vi "Formic Queen.vi"(8 "error in (no error)":errorcluster, 9 "SelfID":i32, 10 "Map":i32[](array[numeric]), 11 "Mother in":refnum<class "Formics.lvclass">) -> (0 "error out":errorcluster, 1 "Direction":T1, 2 "Action":T2, 3 "Mother out":refnum<class "Formics.lvclass">, 4 "Replicated Class":refnum<class "Formics.lvclass">)   [LabVIEW 2015, in "Formics.lvclass"]
uses:
  Formics.lvclass
  Type Defs/Action Enum.ctl
  Type Defs/Direction Enum.ctl
  Formics.lvclass/Formics.ctl
  SquareStatus.ctl
  Formic Types.ctl
  Kamikaze DVR Cluster.ctl
  Type Defs/SB Type Defs.lvlib
  Common/Common.lvlib
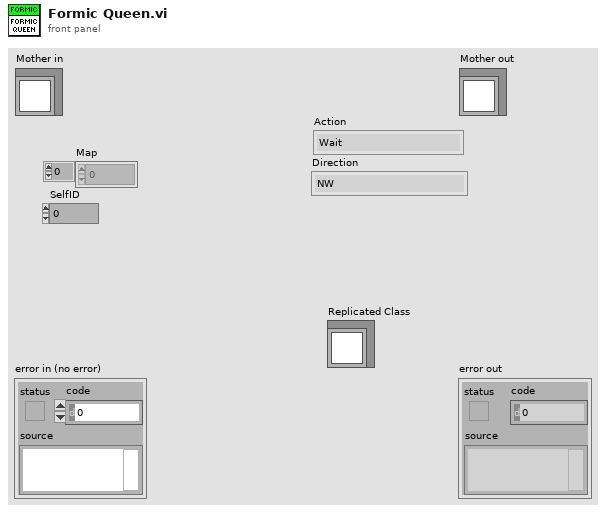
[diagram p1: front panel]
types:
  T1 = typedef "SB Type Defs.lvlib/Direction Enum.ctl" = enum16{"NW", "N", "NE", "E", "SE", "S", "SW", "W"}
  T2 = typedef "SB Type Defs.lvlib/Action Enum.ctl" = enum16{"Wait", "Move", "Attack", "Replicate"}
  T3 = typedef "Kamikaze DVR Cluster.ctl" = cluster{"Kamikaze?":bool, "Direction":u8}
  T4 = typedef "Formics.lvclass/Formic Types.ctl" = enum16{"Queen Bee", "Protector Bee", "Daughter Bee", "Worker Bee", "Coward"}
  T5 = typedef "Formics.lvclass/SquareStatus.ctl" = cluster{"ID":i32, "Heartbeat":bool, "MyPosition":cluster{"X":i32, "Y":i32}}
  T6 = typedef "Formics.lvclass/Kamikaze DVR.ctl" = refnum<data-value>
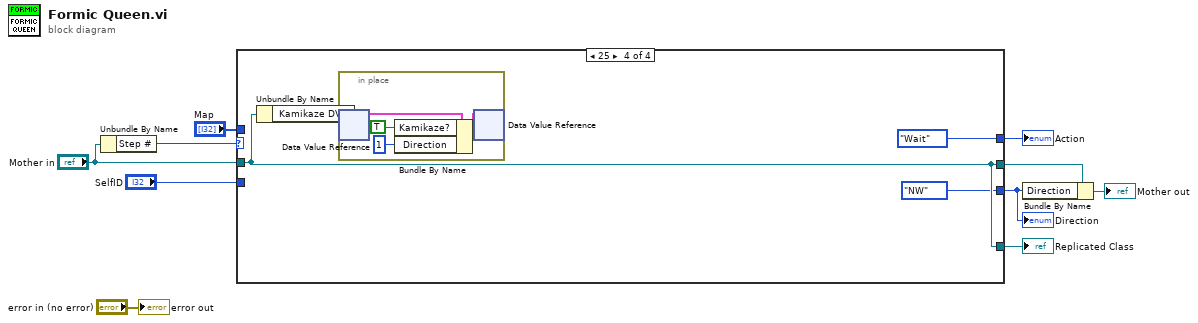
[diagram p0: block diagram]
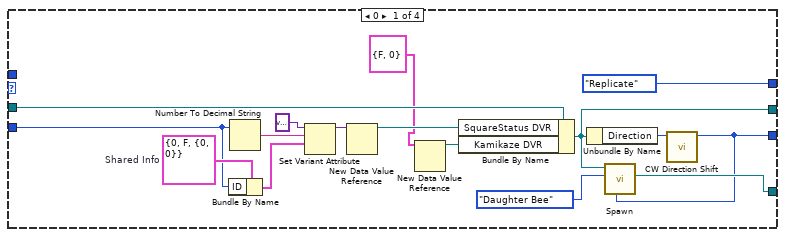
[diagram p2: hidden frame]
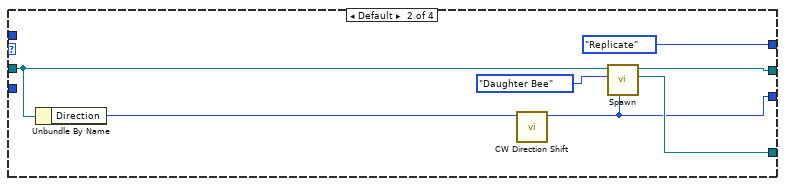
[diagram p3: hidden frame]
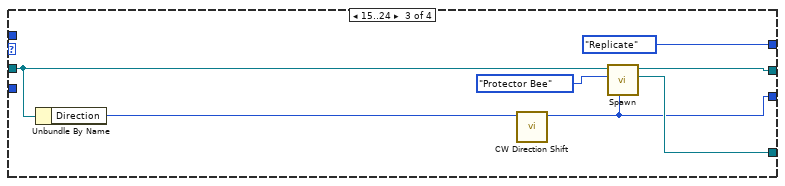
[diagram p4: hidden frame]
diagram:
  n1 = Unbundle By Name("Mother in") -> ("Step #"=w7:i32)
  n2 = case shown="25" w7 {
    tunnel: [w15 w29 w36 w42] -> w9
    tunnel: "Mother in" -> [w20 w30 w37 w42]
    tunnel: "SelfID" -> [w19 _ _ _]
    tunnel: "Map" -> [_ _ _ _]
    tunnel: [Action_Enum."Replicate" ("Action") Action_Enum."Replicate" ("Action") Action_Enum."Replicate" ("Action") Action_Enum."Wait" ("Action")] -> w4
    tunnel: [w14 w28 w35 Direction_Enum."NW" ("Direction")] -> w1
    tunnel: [w17 w31 w38 w42] -> w3
    frame 0 {
      w24 = T5 {"ID"=0, "Heartbeat"=FALSE, "MyPosition"={"X"=0, "Y"=0}}  # Shared Info
      n3 = Bundle By Name(cluster=w24, "ID"=w19) -> (w25:T5)
      n4 = Number To Decimal String(number=w19) -> (decimal integer string=w26:string)  [unwired: 1 in]
      n5 = Set Variant Attribute(Variant=variant ("variant"), name=w26, value=w25) -> (Variant out=w23:variant)  [unwired: 1 in, 2 out]
      n6 = New Data Value Reference(data value=w23) -> (data value reference=w22:refnum<data-value>)  [unwired: 1 in, 1 out]
      n7 = New Data Value Reference(data value=T3 {"Kamikaze?"=FALSE, "Direction"=0}) -> (data value reference=w11:refnum<data-value>)  [unwired: 1 in, 1 out]
      n8 = Bundle By Name(cluster=w20, "SquareStatus DVR"=w22, "Kamikaze DVR"=w11) -> (w15:refnum<class "Formics.lvclass">)
      n9 = Unbundle By Name(w15) -> ("Direction"=w13:i32)
      n10 = call "CW Direction Shift.vi"("Direction"=w13) -> ("Numeric"=w14:i32)  [unwired: 10 in]
      n11 = call "Spawn.vi"("Start Direction"=w14, "Directive"=Formic_Types."Daughter Bee", "Mother in"=w15) -> ("Replicated Class"=w17:refnum<class "Formics.lvclass">)  [unwired: 6 in, 2 out]
    }
    frame Default {
      n12 = Unbundle By Name(w30) -> ("Direction"=w27:i32)
      n13 = call "CW Direction Shift.vi"("Direction"=w27) -> ("Numeric"=w28:i32)  [unwired: 10 in]
      n14 = call "Spawn.vi"("Start Direction"=w28, "Directive"=Formic_Types."Daughter Bee", "Mother in"=w30) -> ("Replicated Class"=w31:refnum<class "Formics.lvclass">, "Mother out"=w29:refnum<class "Formics.lvclass">)  [unwired: 6 in, 1 out]
    }
    frame 15..24 {
      n15 = Unbundle By Name(w37) -> ("Direction"=w34:i32)
      n16 = call "CW Direction Shift.vi"("Direction"=w34) -> ("Numeric"=w35:i32)  [unwired: 10 in]
      n17 = call "Spawn.vi"("Start Direction"=w35, "Directive"=Formic_Types."Protector Bee", "Mother in"=w37) -> ("Replicated Class"=w38:refnum<class "Formics.lvclass">, "Mother out"=w36:refnum<class "Formics.lvclass">)  [unwired: 6 in, 1 out]
    }
    frame 25 {
      n18 = Unbundle By Name(w42) -> ("Kamikaze DVR"=w44:T6)
      n19 = in-place {
        n20 = in-place-dvr #1(w44) -> (w48:T3)  [unwired: 1 out]
        n21 = Bundle By Name(cluster=w48, "Kamikaze?"=TRUE, "Direction"=u8 1) -> (w47:T3)
        n22 = in-place-dvr #1(w47) -> ()  [unwired: 2 out]
      }
    }
  }
  "Action" <- w4
  "Direction" <- w1
  "Replicated Class" <- w3
  n23 = Bundle By Name(cluster=w9, "Direction"=w1) -> (→"Mother out":refnum<class "Formics.lvclass">)
  "error out" <- "error in (no error)"
